vi "thermo_get_result_stats.vi"(7 "temp channel":T1[][](array[typedef])) -> (1 "temp max":dbl format="%0.2f", 2 "RH max":dbl format="%0.2f", 3 "pres max":dbl format="%0.2f", 6 "temp ua":dbl format="%0.2f", 8 "RH ua":dbl format="%0.2f", 10 "pres ua":dbl format="%0.2f", 12 "temp min":dbl format="%0.2f", 13 "RH min":dbl format="%0.2f", 14 "pres min":dbl format="%0.2f")   [LabVIEW 2020]
uses:
  thermo_read.ctl
  varilib/varilib.lvlib
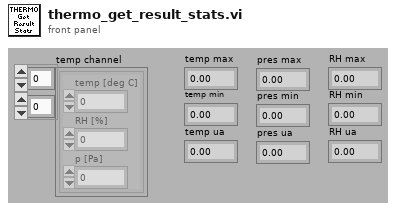
[diagram p1: front panel]
types:
  T1 = typedef "thermo_read.ctl" = cluster{"temp [deg C]":dbl, "RH [%]":dbl, "p [Pa]":dbl}
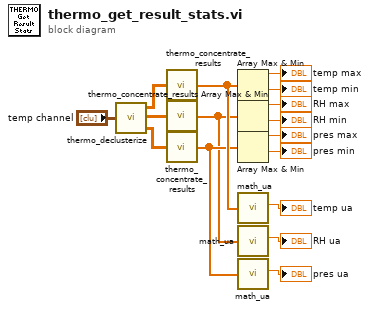
[diagram p0: block diagram]
diagram:
  n1 = call "thermo_declusterize.vi"("temp channel"="temp channel") -> ("temperature"=w6:dbl[][], "RH"=w5:dbl[][], "pressure"=w4:dbl[][])
  n2 = call "thermo_concentrate_results.vi"("array in"=w6) -> ("vector out"=w3:dbl[])
  n3 = call "thermo_concentrate_results.vi"("array in"=w5) -> ("vector out"=w1:dbl[])
  n4 = call "thermo_concentrate_results.vi"("array in"=w4) -> ("vector out"=w2:dbl[])
  n5 = Array Max & Min(array=w3) -> (max value=→"temp max":dbl, min value=→"temp min":dbl)  [unwired: 2 out]
  n6 = Array Max & Min(array=w1) -> (max value=→"RH max":dbl, min value=→"RH min":dbl)  [unwired: 2 out]
  n7 = Array Max & Min(array=w2) -> (max value=→"pres max":dbl, min value=→"pres min":dbl)  [unwired: 2 out]
  n8 = call "math_ua.vi"("x"=w3) -> ("ua(x)"=→"temp ua":dbl)  [unwired: 3 out]
  n9 = call "math_ua.vi"("x"=w1) -> ("ua(x)"=→"RH ua":dbl)  [unwired: 3 out]
  n10 = call "math_ua.vi"("x"=w2) -> ("ua(x)"=→"pres ua":dbl)  [unwired: 3 out]
